vi "Primary Pressure Balance.vi"(0 "MHX Length":dbl, 1 "Pipe Diameter":dbl, 2 "MHX Tube Diameter":dbl, 3 "Pri Loop Height":dbl, 4 "RX Height":dbl, 5 "Primary Average Density":dbl, 6 "Pri Loop Width":dbl, 8 "Thermal Driving Pressure":dbl, 9 "Primary Hot Density":dbl, 10 "AC Friction Factor":dbl, 11 "Primary Cold Density":dbl, 12 "CD Friction Factor":dbl, 13 "Core Channel Equivalent Diameter":dbl, 14 "DF Friction Factor":dbl, 15 "Downcomer Gap":dbl, 16 "FG Friction Factor":dbl, 17 "MHX Velocity":dbl, 18 "GA Friction Factor":dbl, 19 "Hot Leg Velocity":dbl, 26 "RX Velocity":dbl, 27 "Cold Leg Velocity":dbl) -> (20 "Elbow Loss":dbl, 21 "Pressure Balance (Pa)":dbl, 22 "Pipe Loss":dbl, 23 "MHX Loss":dbl, 24 "RX Loss":dbl)   [LabVIEW 2019]
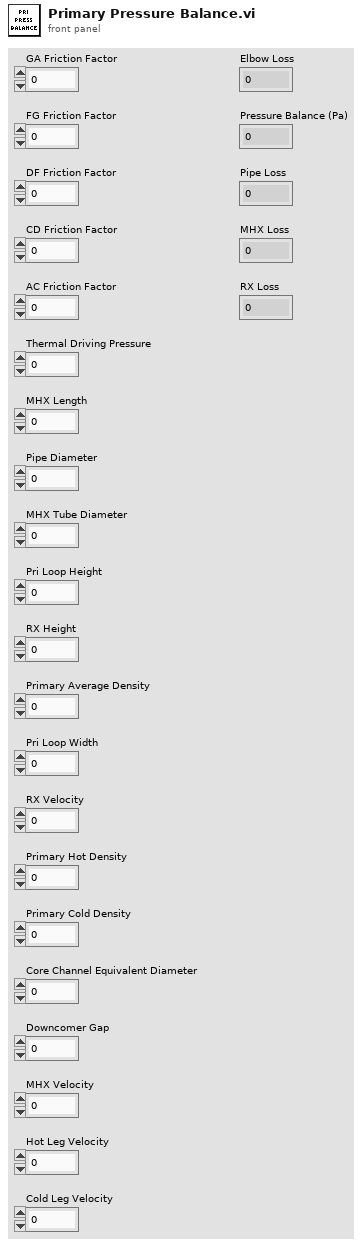
[diagram p1: front panel]
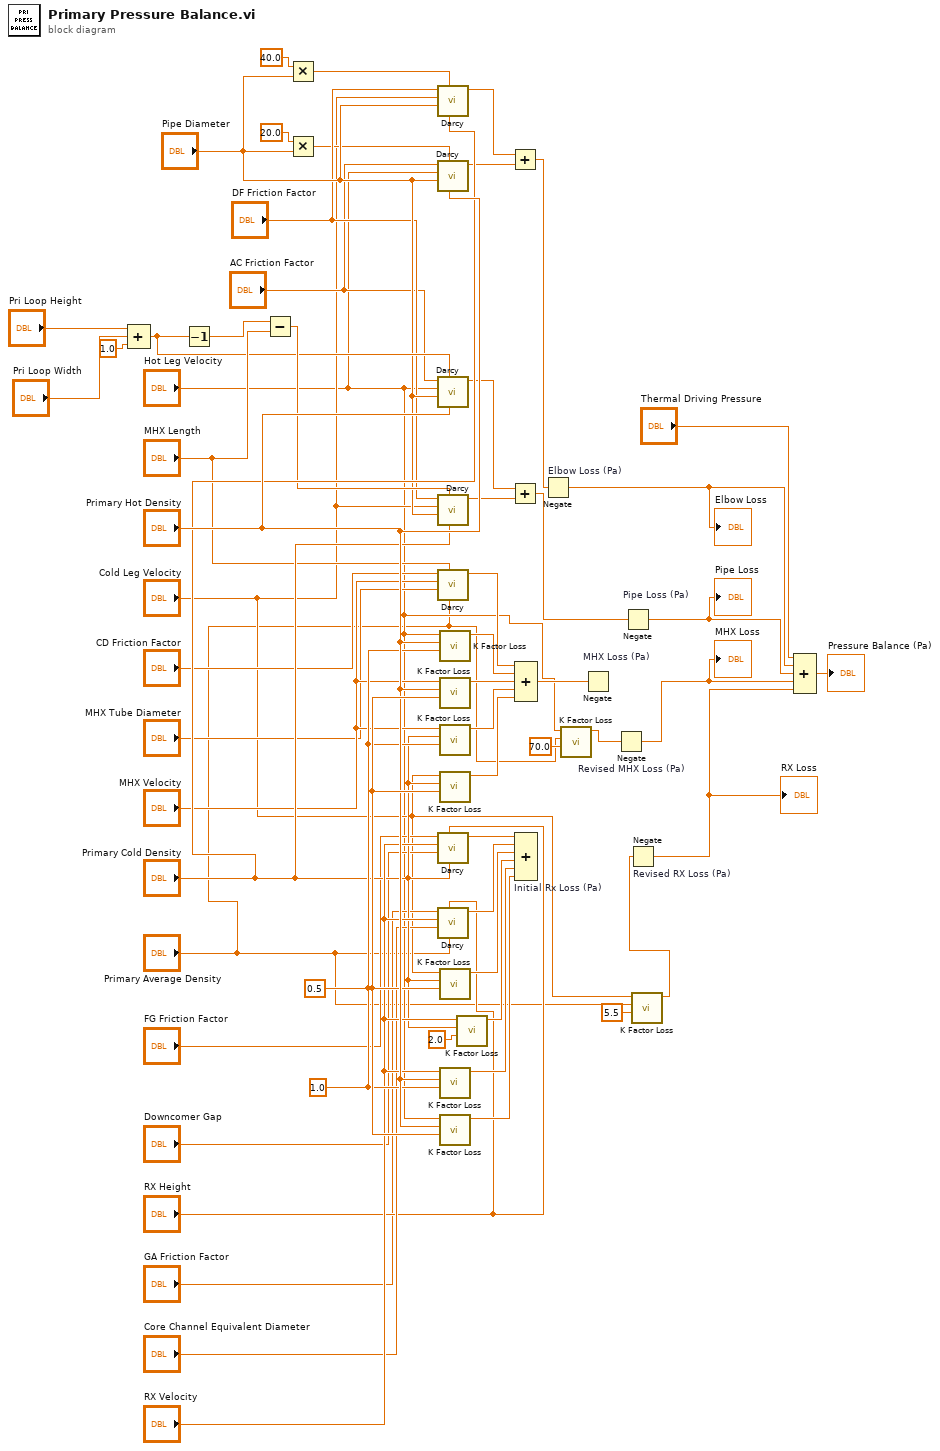
[diagram p0: block diagram]
diagram:
  w51 = 0.5 ("K")
  w49 = 1.0 ("K")
  n1 = Compound Arithmetic op=ADD("Pri Loop Height", "Pri Loop Width", 1.0 ("value")) -> (w22:dbl)
  n2 = Decrement(x=w22) -> (x-1=w23:dbl)
  n3 = Subtract(x=w23, y="MHX Length") -> (x-y=w24:dbl)
  n4 = Multiply(x=40.0, y="Pipe Diameter") -> (x*y=w12:dbl)
  n5 = Multiply(x=20.0, y="Pipe Diameter") -> (x*y=w9:dbl)
  n6 = call "Darcy.vi"("Density (kg/m^3)"="Primary Cold Density", "Length (m)"=w12, "Effective Diameter (m)"="Pipe Diameter", "Velocity (m/s)"="Cold Leg Velocity", "Friction Factor"="DF Friction Factor") -> ("Loss (Pa)"=w14:dbl)  [unwired: 6 in]
  n7 = call "Darcy.vi"("Density (kg/m^3)"="Primary Hot Density", "Length (m)"=w9, "Effective Diameter (m)"="Pipe Diameter", "Velocity (m/s)"="Hot Leg Velocity", "Friction Factor"="AC Friction Factor") -> ("Loss (Pa)"=w13:dbl)  [unwired: 6 in]
  n8 = call "Darcy.vi"("Density (kg/m^3)"="Primary Hot Density", "Length (m)"=w22, "Effective Diameter (m)"="Pipe Diameter", "Velocity (m/s)"="Hot Leg Velocity", "Friction Factor"="AC Friction Factor") -> ("Loss (Pa)"=w26:dbl)  [unwired: 6 in]
  n9 = call "Darcy.vi"("Density (kg/m^3)"="Primary Cold Density", "Length (m)"=w24, "Effective Diameter (m)"="Pipe Diameter", "Velocity (m/s)"="Cold Leg Velocity", "Friction Factor"="DF Friction Factor") -> ("Loss (Pa)"=w27:dbl)  [unwired: 6 in]
  n10 = call "Darcy.vi"("Density (kg/m^3)"="Primary Average Density", "Length (m)"="MHX Length", "Effective Diameter (m)"="MHX Tube Diameter", "Velocity (m/s)"="MHX Velocity", "Friction Factor"="CD Friction Factor") -> ("Loss (Pa)"=w35:dbl)  [unwired: 6 in]
  n11 = call "Darcy.vi"("Density (kg/m^3)"="Primary Cold Density", "Length (m)"="RX Height", "Effective Diameter (m)"="Downcomer Gap", "Velocity (m/s)"="RX Velocity", "Friction Factor"="FG Friction Factor") -> ("Loss (Pa)"=w52:dbl)  [unwired: 6 in]
  n12 = call "Darcy.vi"("Density (kg/m^3)"="Primary Average Density", "Length (m)"="RX Height", "Effective Diameter (m)"="Core Channel Equivalent Diameter", "Velocity (m/s)"="RX Velocity", "Friction Factor"="GA Friction Factor") -> ("Loss (Pa)"=w53:dbl)  [unwired: 6 in]
  n13 = call "K Factor Loss.vi"("K"=w49, "Density (kg/m^3)"="Primary Hot Density", "Velocity (m/s)"="Hot Leg Velocity") -> ("Loss (Pa)"=w36:dbl)  [unwired: 8 in]
  n14 = call "K Factor Loss.vi"("K"=w51, "Density (kg/m^3)"="Primary Hot Density", "Velocity (m/s)"="MHX Velocity") -> ("Loss (Pa)"=w37:dbl)  [unwired: 8 in]
  n15 = call "K Factor Loss.vi"("K"=w49, "Density (kg/m^3)"="Primary Cold Density", "Velocity (m/s)"="MHX Velocity") -> ("Loss (Pa)"=w38:dbl)  [unwired: 8 in]
  n16 = call "K Factor Loss.vi"("K"=w51, "Density (kg/m^3)"="Primary Cold Density", "Velocity (m/s)"="Cold Leg Velocity") -> ("Loss (Pa)"=w39:dbl)  [unwired: 8 in]
  n17 = call "K Factor Loss.vi"("K"=w49, "Density (kg/m^3)"="Primary Cold Density", "Velocity (m/s)"="Cold Leg Velocity") -> ("Loss (Pa)"=w54:dbl)  [unwired: 8 in]
  n18 = call "K Factor Loss.vi"("K"=w49, "Density (kg/m^3)"="Primary Hot Density", "Velocity (m/s)"="RX Velocity") -> ("Loss (Pa)"=w56:dbl)  [unwired: 8 in]
  n19 = call "K Factor Loss.vi"("K"=w51, "Density (kg/m^3)"="Primary Hot Density", "Velocity (m/s)"="Hot Leg Velocity") -> ("Loss (Pa)"=w57:dbl)  [unwired: 8 in]
  n20 = call "K Factor Loss.vi"("K"=2.0, "Density (kg/m^3)"="Primary Cold Density", "Velocity (m/s)"="RX Velocity") -> ("Loss (Pa)"=w55:dbl)  [unwired: 8 in]
  n21 = Add(x=w14, y=w13) -> (x+y=w15:dbl)
  n22 = Add(x=w26, y=w27) -> (x+y=w25:dbl)
  n23 = Compound Arithmetic op=ADD(w35, w36, w37, w38, w39) -> (w40:dbl)
  n24 = Compound Arithmetic op=ADD "Initial Rx Loss (Pa)"(w52, w53, w54, w55, w56, w57) -> ()  [unwired: 1 out]
  n25 = Negate "Elbow Loss (Pa)"(x=w15) -> (-x=w29:dbl)
  "Elbow Loss" <- w29
  n26 = call "K Factor Loss.vi"("K"=70.0, "Density (kg/m^3)"="Primary Average Density", "Velocity (m/s)"="Hot Leg Velocity") -> ("Loss (Pa)"=w2:dbl)  [unwired: 8 in]
  n27 = Negate "MHX Loss (Pa)"(x=w40) -> ()  [unwired: 1 out]
  n28 = Negate "Revised MHX Loss (Pa)"(x=w2) -> (-x=w1:dbl)
  "MHX Loss" <- w1
  n29 = Negate "Pipe Loss (Pa)"(x=w25) -> (-x=w30:dbl)
  "Pipe Loss" <- w30
  n30 = call "K Factor Loss.vi"("K"=5.5, "Density (kg/m^3)"="Primary Average Density", "Velocity (m/s)"="Cold Leg Velocity") -> ("Loss (Pa)"=w6:dbl)  [unwired: 8 in]
  n31 = Negate "Revised RX Loss (Pa)"(x=w6) -> (-x=w58:dbl)
  "RX Loss" <- w58
  n32 = Compound Arithmetic op=ADD("Thermal Driving Pressure", w29, w30, w1, w58) -> (→"Pressure Balance (Pa)":dbl)
